vi "Create_PDF4Box.vi"(0 "Tableau de valves":string[](array[string])=["112105740008010001", "112105740008010002", "112105740008010003", "112105740008010004", "112105740008010005", "112105740008010006", "112105740008010007", "112105740008010008", "112105740008010009", "112105740008010010", "112105740008010011", "112105740008010012", "112105740008010013", "112105740008010014", "112105740008010015", "112105740008010016", "112105740008010017", "112105740008010018", "112105740008010019", "112105740008010020", "112105740008010021", "112105740008010022", "112105740008010023", "112105740008010024", "112105740008010025"], 1 "Produit":string="12-216C-04521 EQIFIL 417mA 14.4ohm", 2 "Client":string="EMS Electro Medical System", 3 "Nombre Cartons":string="4", 4 "Numero Carton":string="1", 5 "Cust_Prod_Ref":string="EL-360", 6 "Cust_Indice":string="03", 7 "error in (no error)":errorcluster caption="entrée d'erreur (pas d'erreur)", 8 "Commande":string="03838/08-01.07.01", 9 "Cust_Order":string="CF-08-0253/2") -> (27 "error out":errorcluster caption="sortie d'erreur")   [LabVIEW 2020]
doc: "Le fichier modèle (BoxFile.txt) pour le générateur de PDF doit se trouver dans le répertoire:\n\\data\\pydist\nLe PDF généré pour le carton se trouve aussi dans ce répertoire après sa création\nL'executable python pour la génération du PDF se trouve dans ce même répertoire,\nl'appel de ce générateur se fait avec la ligne de commande : \n\\data\\pydist\\Create_Cust_PDF4Box.exe\nPour l'instrant l'éxécutable Python ne gère qu'1 feuille PDF pouvant contenir au maximum\n40 codes barre, à modifier si nécessaire (pas plus de 25/box selon CDC...)"
uses:
  <vilib>/Utility/NIReport.llb/NI_ReportGenerationCore.lvlib
panel:
  out "standard output (Batch)":string caption="sortie standard"
  out "standard error (Batch)":string caption="erreur standard"
  out "return code (Batch)":i32 caption="code de retour"
  out "default printer":string caption="imprimante par défaut"
  out "system configured printers":string[](array[string]) caption="imprimantes système configurées"
  in  "Nom de l'executable":string="Create_Cust_PDF4Box.exe"
  # "FONCTIONNEMENT OK :\nVoir les commentaires du script\n\"PDF2printer.bat\" pour explications.\nEn cas de changement du fonctionnement,\non peut agir directement avec ce script sur\ncertains paramêtres."
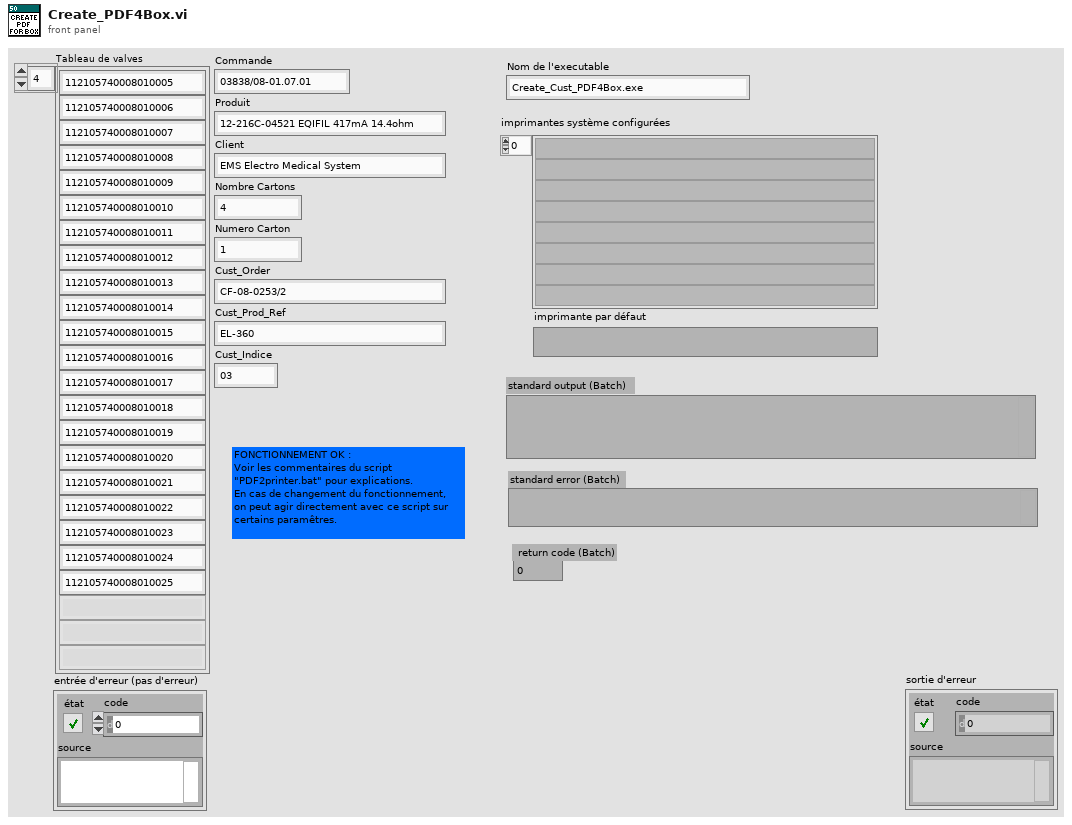
[diagram p1: front panel]
types:
  T1 = enum16{"open", "replace", "create", "open or create", "replace or create", "replace or create with confirmation"}
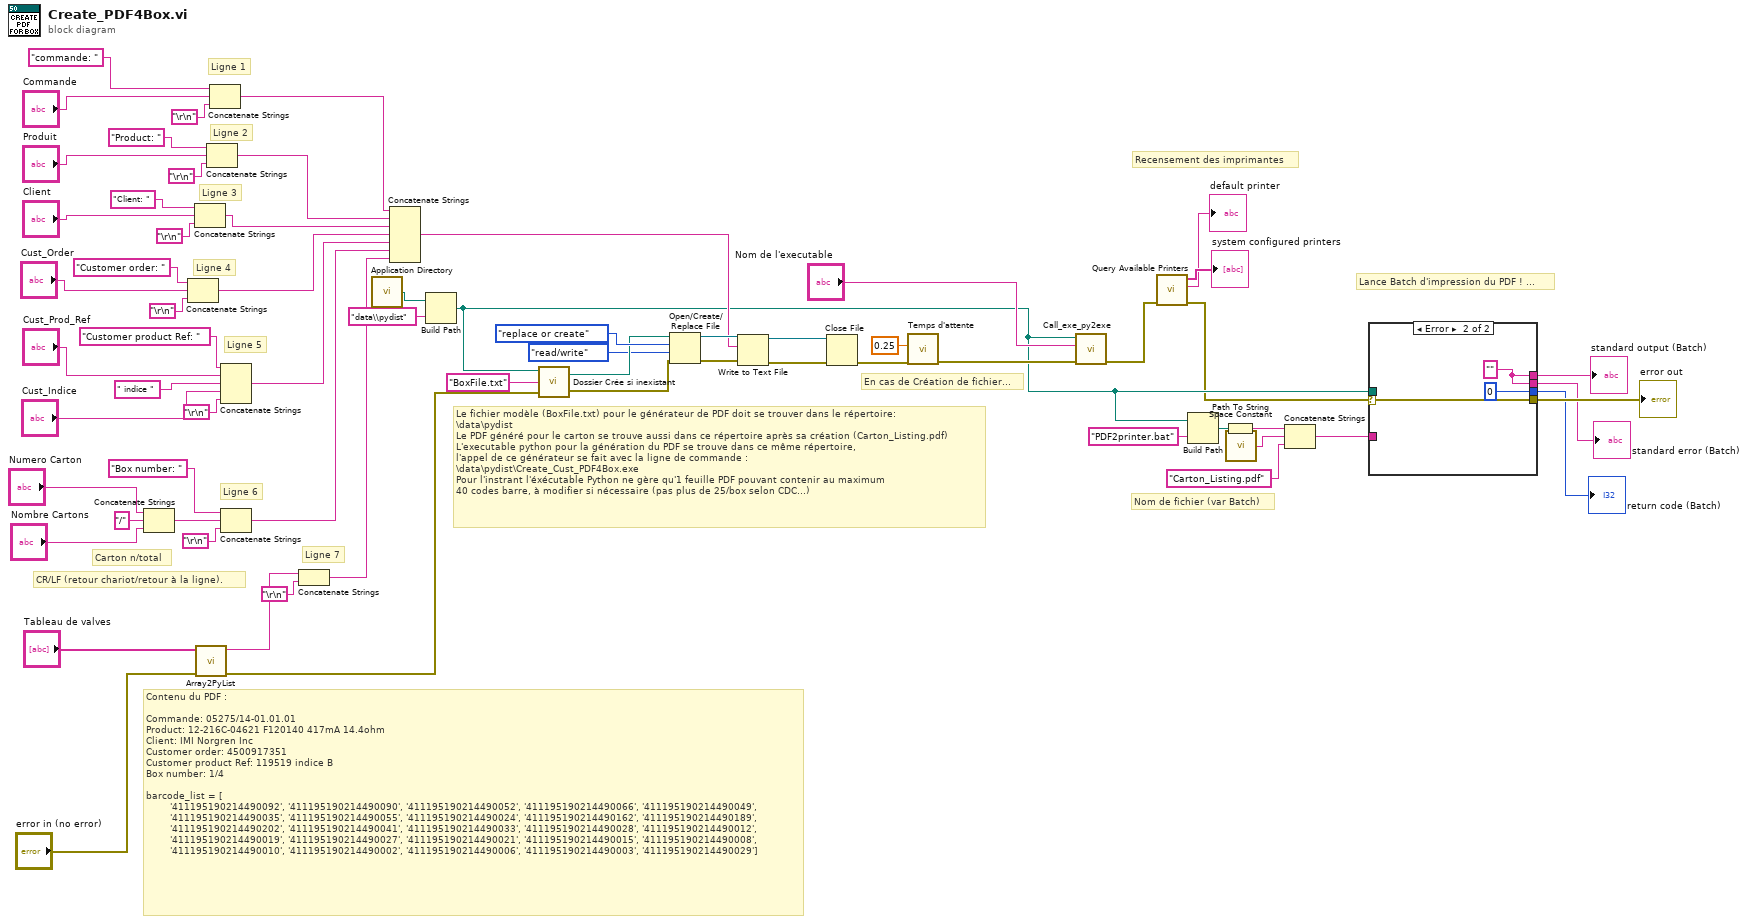
[diagram p0: block diagram]
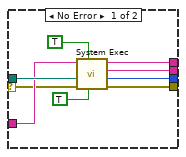
[diagram p2: hidden frame]
diagram:
  # "Nom de fichier (var Batch)"
  # "Recensement des imprimantes"
  # "Lance Batch d'impression du PDF ! ..."
  # "En cas de Création de fichier..."
  # "Le fichier modèle (BoxFile.txt) pour le générateur de PDF doit se trouver dans le répertoire:\n\\data\\pydist\nLe PDF généré pour le carton se trouve aussi dans ce répertoire après sa création (Carton_Listing.pdf)\nL'executable python pour la génération du PDF se trouve dans ce même répertoire,\nl'appel de ce générateur se fait avec la ligne de commande : \n\\data\\pydist\\Create_Cust_PDF4Box.exe\nPour l'instrant l'éxécutable Python ne gère qu'1 feuille PDF pouvant contenir au maximum\n40 codes barre, à modifier si nécessaire (pas plus de 25/box selon CDC...)"
  # "Ligne 7"
  # "Ligne 6"
  # "Ligne 5"
  # "Ligne 4"
  # "Ligne 3"
  # "Ligne 2"
  # "Ligne 1"
  # "CR/LF (retour chariot/retour à la ligne)."
  # "Carton n/total"
  # "Contenu du PDF : \n\nCommande: 05275/14-01.01.01\nProduct: 12-216C-04621 F120140 417mA 14.4ohm\nClient: IMI Norgren Inc\nCustomer order: 4500917351\nCustomer product Ref: 119519 indice B\nBox number: 1/4\n\nbarcode_list = [\n        '411195190214490092', '411195190214490090', '411195190214490052', '411195190214490066', '411195190214490049',\n        '411195190214490035', '411195190214490055', '411195190214490024', '411195190214490162', '411195190214490189',\n        '411195190214490202', '411195190214490041', '411195190214490033', '411195190214490028', '411195190214490012',\n        '411195190214490019', '411195190214490027', '411195190214490021', '411195190214490015', '411195190214490008',\n        '411195190214490010', '411195190214490002', '411195190214490006', '411195190214490003', '411195190214490029']"
  n1 = Concatenate Strings("Numero Carton", "/", "Nombre Cartons") -> (w60:string)
  n2 = Concatenate Strings("Customer order: ", "Cust_Order", "\r\n") -> (w29:string)
  n3 = Concatenate Strings("Client: ", "Client", "\r\n") -> (w30:string)
  n4 = call "Array2PyList.vi"("error in (no error)"="error in (no error)", "Tableau de valves"="Tableau de valves") -> ("error out"=w33:errorcluster, "List_Valves"=w39:string)  [unwired: 8 in]
  n5 = Concatenate Strings("Product: ", "Produit", "\r\n") -> (w31:string)
  n6 = Concatenate Strings("commande: ", "Commande", "\r\n") -> (w32:string)
  n7 = Concatenate Strings("Customer product Ref: ", "Cust_Prod_Ref", " indice ", "Cust_Indice", "\r\n") -> (w28:string)
  n8 = Concatenate Strings("Box number: ", w60, "\r\n") -> (w27:string)
  n9 = Concatenate Strings(w39, "\r\n") -> (w26:string)
  n10 = call <vilib>:"Application Directory.vi"() -> ("Application Directory"=w20:path)
  n11 = Concatenate Strings(w32, w31, w30, w29, w28, w27, w26) -> (w25:string)
  n12 = Build Path(base path=w20, name or relative path="data\\pydist" ("nom ou chemin relatif")) -> (appended path=w9:path)
  n13 = call "Dossier Crée si inexistant.vi"("error in"=w33, "nom sous dossier"="BoxFile.txt" ("nom fichier"), "chemin du dossier IN"=w9) -> ("error out"=w24:errorcluster, "chemin sous dossier OUT"=w38:path)
  n14 = Open/Create/Replace File(file path (use dialog)=w38, error in=w24, operation (0:open)=T1."replace or create" ("opération (0 : open)"), access (0:read/write)=enum16{"read/write", "read-only", "write-only"}."read/write" ("accès (0 : read/write)")) -> (refnum out=w37:refnum<file>, error out=w36:errorcluster)  [unwired: 2 in, 1 out]
  n15 = Write to Text File(file (use dialog)=w37, text=w25, error in=w36) -> (refnum out=w34:refnum<file>, error out=w35:errorcluster)  [unwired: 1 in, 1 out]
  n16 = Close File(refnum=w34, error in=w35) -> (error out=w17:errorcluster)  [unwired: 1 out]
  n17 = call "Temps d'attente"("error in (no error)"=w17, "Delay Time (s)"=0.25) -> ("error out"=w16:errorcluster)  [unwired: 9 in]
  n18 = call "Call_exe_py2exe.vi"("error in (no error)"=w16, "Nom de l'executable"="Nom de l'executable", "Répertoire de travail"=w9) -> ("error out"=w13:errorcluster)  [unwired: 8 in]
  n19 = call <vilib>:"Query Available Printers.vi"("error in (no error)"=w13) -> ("error out"=w1:errorcluster, "default printer"=→"default printer":string, "system configured printers"=→"system configured printers":string[])  [unwired: 8 in]
  n20 = Build Path(base path=w9, name or relative path="PDF2printer.bat" ("nom ou chemin relatif")) -> (appended path=w11:path)
  n21 = Path To String(path=w11) -> (string=w10:string)
  n22 = call <vilib>:"Space Constant.vi"() -> ("String"=w7:string)
  n23 = Concatenate Strings(w10, w7, "Carton_Listing.pdf" ("nom fichier")) -> (w8:string)
  n24 = case shown="Error" w1 {
    selector: w1 -> [w67 w78]
    tunnel: w9 -> [w74 _]
    tunnel: w8 -> [w73 _]
    tunnel: [w72 w78] -> w5
    tunnel: [w71 0 ("return code")] -> w4
    tunnel: [w70 w76] -> w3
    tunnel: [w69 w76] -> w2
    frame No Error {
      n25 = call <vilib>:"System Exec.vi"("run minimized? (F)"=TRUE, "wait until completion? (T)"=TRUE, "error in (no error)"=w67, "working directory"=w74, "command line"=w73) -> ("error out"=w72:errorcluster, "return code"=w71:i32, "standard error"=w70:string, "standard output"=w69:string)  [unwired: 3 in]
    }
    frame Error {
      w76 = "" ("standard error")
    }
  }
  "error out" <- w5
  "return code (Batch)" <- w4
  "standard error (Batch)" <- w3
  "standard output (Batch)" <- w2
